vi "FPGA_CurrentSampling.vi"() -> ()   [LabVIEW 2014]
uses:
  <vilib>/rvi/Emulation/niFpgaGetClockAttributes.vi
  <vilib>/rvi/Emulation/niFpgaSctlEmulationGetInTimedLoop.vi
  <vilib>/rvi/Emulation/niFpgaEmulationReportErrorSimple.vi
  <vilib>/rvi/eio/common/nirviEmuTemplateMethod_errors.vi
  <vilib>/rvi/interface/RandomDataEmulation/niFpgaRandomDataHandleErrors.vi
  <vilib>/rvi/Emulation/niFpgaCriticalErrorInLSC.vi
  <vilib>/eio/EIONode/EIONode.xnode
  <vilib>/rvi/DataTransferAndStorage/Container/XNode/niFpgaContainer.xnode
  <vilib>/rvi/interface/RandomDataEmulation/nirviRandomDataFpgaReadWriteTemplate.vi
panel:
  in  "Count(uSec)":u32=20
  out "Stopped?":bool
  out "PresNum":i32
  in  "stop":bool
  in  "SampleNum":i32
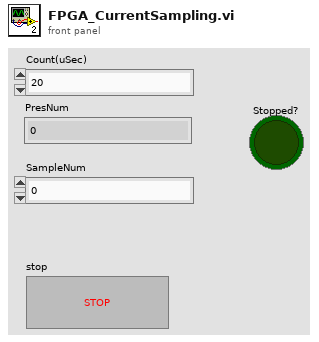
[diagram p1: front panel]
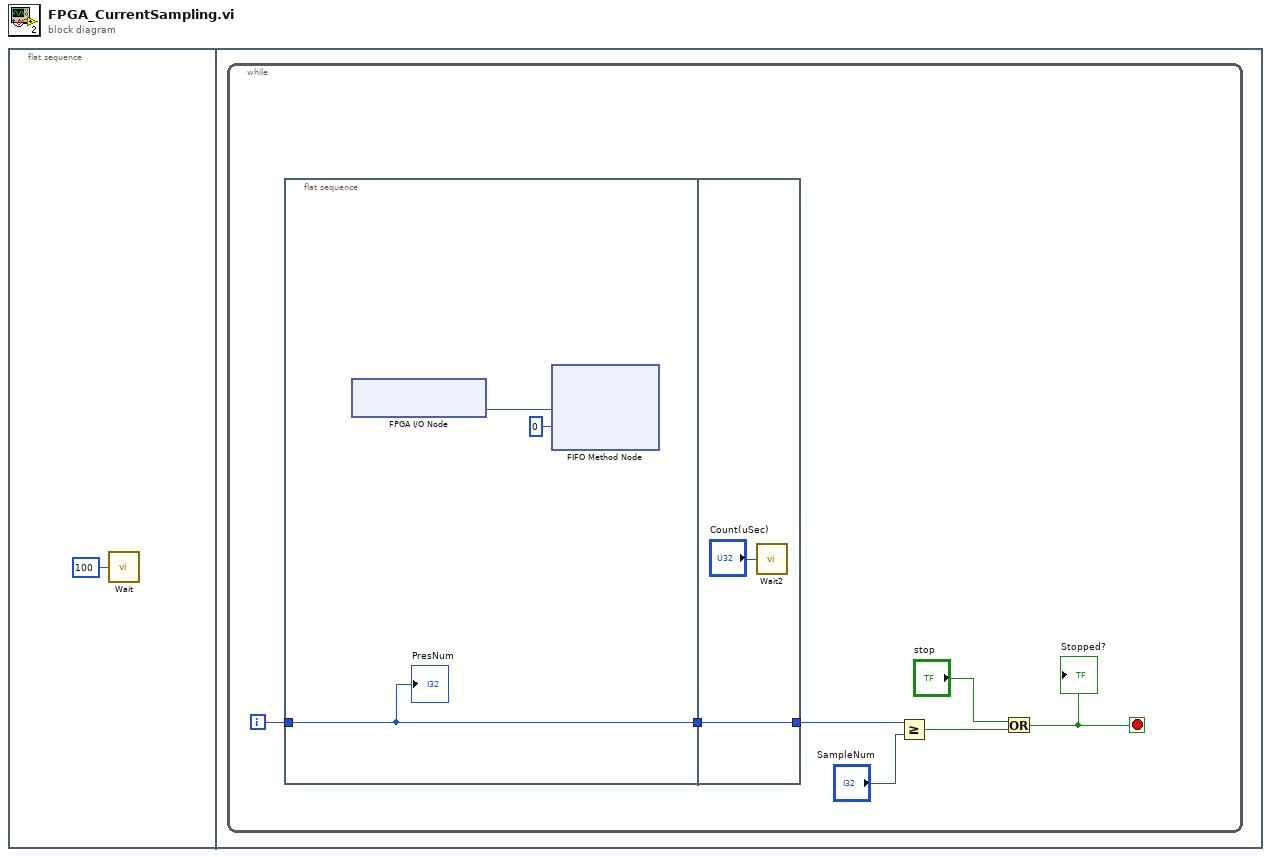
[diagram p0: block diagram]
diagram:
  n1 = flat-sequence {
    frame #0 {
      n2 = call "Wait"("Count(mSec)"=u32 100 ("Count(uSec)")) -> ()  [unwired: 1 out]
    }
    frame #1 {
      n3 = while {
        i -> [w8]
        stop <- w4 stop-if-true
        n4 = flat-sequence {
          tunnel: w8 -> [w9]
          tunnel: [w9] -> w7
          tunnel: w7 -> [w12]
          tunnel: [w12] -> w6
          frame #0 {
            n5 = xnode "FPGA I/O Node"() -> ("Connector0/AI1"=w11:i16)  [unwired: 1 in, 1 out]
            n6 = xnode ("FIFO Method Node")("Element"=w11, "Timeout"=0) -> ()  [unwired: 1 in, 2 out]
            "PresNum" <- w9
          }
          frame #1 {
            n7 = call "Wait2"("Count(uSec)"="Count(uSec)") -> ()  [unwired: 1 out]
          }
        }
        n8 = Greater Or Equal?(x=w6, y="SampleNum") -> (x >= y?=w3:bool)
        n9 = Or(x="stop", y=w3) -> (x .or. y?=w4:bool)
        "Stopped?" <- w4
      }
    }
  }
